vi "VIPM Uninstall All VI Packages By Name.vi"   [LabVIEW 2016, in "Script.lvlib"]
uses:
  Script.lvlib
  <vilib>/Wiresmith Technology/G CLI/Argument Parser/Option Class/Option Configuration.ctl
  <vilib>/Wiresmith Technology/G CLI/Argument Parser/Option Class/Argument Type.ctl
  <vilib>/Wiresmith Technology/G CLI/CLI Class/CLI.lvclass
  <vilib>/Wiresmith Technology/G CLI/Argument Parser/Option Class/Option.lvclass
  <vilib>/Wiresmith Technology/G CLI/Argument Parser/Option Set Class/Option Set.lvclass
  <vilib>/JKI/VIPM API/VIPM API_vipm_api.lvlib
types:
  T1 = typedef "Option Parser.lvlib/Option.lvclass/Option Configuration.ctl" = cluster{"Option Type":T2, "Option Labels":string[], "Key":string, "Description":string, "Required":bool, "Default Value":string}
  T2 = typedef "Option Parser.lvlib/Option.lvclass/Argument Type.ctl" = enum16{"flag", "value"}
  T3 = typedef "VIPM API_vipm_api.lvlib/Library Contents Cluster_vipm_api.ctl" = cluster{"Package Name":string, "Version":string, "Display Name":string, "Repository Name":string, "Company Name":string, "License Type":string, "Installed":bool, "Deprecated":bool, "Dependency or Conflict Problem":bool, "Downloaded":bool}
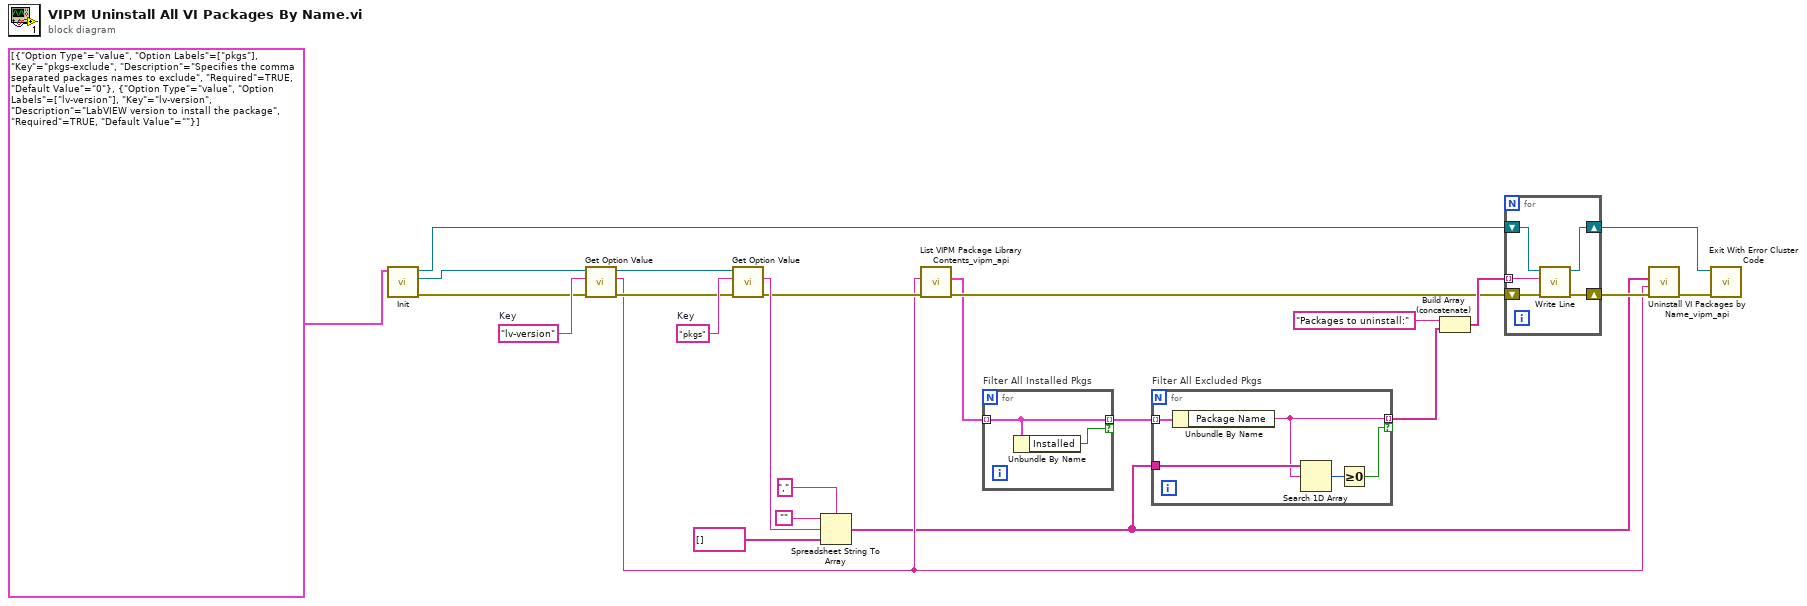
[diagram p0: block diagram]
diagram:
  w18 = "lv-version"  # Key
  w24 = "pkgs"  # Key
  n1 = call "Init.vi"("Options"=T1[] [{"Option Type"=enum."value", "Option Labels"=["pkgs"], "Key"="pkgs-exclude", "Description"="Specifies the comma separated packages names to exclude", "Required"=TRUE, "Default Value"="0"}, {"Option Type"=enum."value", "Option Labels"=["lv-version"], "Key"="lv-version", "Description"="LabVIEW version to install the package", "Required"=TRUE, "Default Value"=""}]) -> ("error out"=w11:errorcluster, "Option Set out"=w10:refnum<class "Option Set.lvclass">, "CLI out"=w9:refnum<class "CLI.lvclass">)  [unwired: 8 in]
  n2 = call <vilib>:"Get Option Value.vi"("error in (no error)"=w11, "Option Key"=w18, "Option Set in"=w10) -> ("error out"=w17:errorcluster, "Value"=w5:string, "Option Set out"=w16:refnum<class "Option Set.lvclass">)  [unwired: 5 in, 1 out]
  n3 = call <vilib>:"Get Option Value.vi"("error in (no error)"=w17, "Option Key"=w24, "Option Set in"=w16) -> ("error out"=w7:errorcluster, "Value"=w15:string)  [unwired: 5 in, 2 out]
  n4 = Spreadsheet String To Array(delimiter (Tab)=",", format string="", spreadsheet string=w15, array type (2D Dbl)=string[] [] ("Value")) -> (array=w2:string[])
  n5 = call <vilib>:"List VIPM Package Library Contents_vipm_api.vi"("error in (no error)"=w7, "LabVIEW Version"=w5) -> ("error out"=w6:errorcluster, "Library Contents []"=w4:T3[])  [unwired: 7 in, 1 out]
  n6 = for "Filter All Installed Pkgs" {
    tunnel: w4 -> [w26] mode=indexing
    tunnel: [w26] -> w3 mode=indexing if=w25
    n7 = Unbundle By Name(w26) -> ("Installed"=w25:bool)
  }
  n8 = for "Filter All Excluded Pkgs" {
    tunnel: w3 -> [w31] mode=indexing
    tunnel: [w27] -> w1 mode=indexing if=w28
    tunnel: w2 -> [w30]
    n9 = Unbundle By Name(w31) -> ("Package Name"=w27:string)
    n10 = Search 1D Array(1D array=w30, element=w27) -> (index of element=w29:i32)  [unwired: 1 in]
    n11 = Greater Or Equal To 0?(x=w29) -> (x >= 0?=w28:bool)
  }
  n12 = Build Array (concatenate)("Packages to uninstall:" ("delimiter (Tab)"), w1) -> (w12:string[])
  n13 = for {
    shift-right: [w34] -> w21
    shift-left: w9 -> [w36]
    shift-right: [w35] -> w23
    shift-left: w6 -> [w33]
    tunnel: w12 -> [w32] mode=indexing
    n14 = call <vilib>:"Write Line.vi"("error in (no error)"=w33, "Text to Write"=w32, "CLI in"=w36) -> ("error out"=w35:errorcluster, "CLI out"=w34:refnum<class "CLI.lvclass">)  [unwired: 7 in]
  }
  n15 = call <vilib>:"Uninstall VI Packages by Name_vipm_api.vi"("error in (no error)"=w23, "LabVIEW Version"=w5, "Package Names to Uninstall []"=w2) -> ("error out"=w22:errorcluster)  [unwired: 8 in]
  n16 = call <vilib>:"Exit With Error Cluster Code.vi"("error in (no error)"=w22, "CLI in"=w21) -> ()  [unwired: 9 in, 1 out]
